vi "BCD码至十进制转换.vi"(9 "低位":u16 format="%x", 11 "高位":u16 format="%x") -> (2 "十进制数":u16)   [LabVIEW 2010]
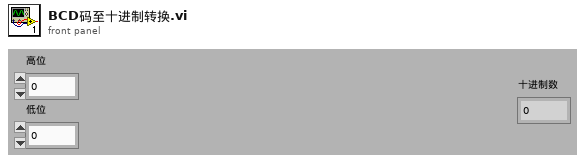
[diagram p1: front panel]
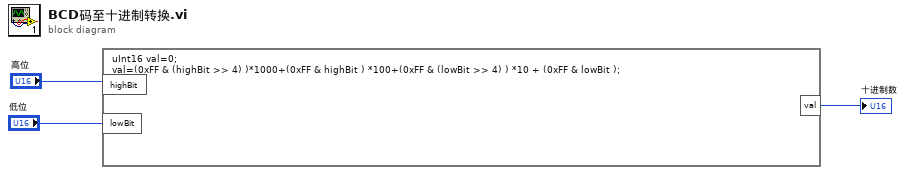
[diagram p0: block diagram]
diagram:
  n1 = formula code="uInt16 val=0;\nval=(0xFF & (highBit >> 4) )*1000+(0xFF & highBit ) *100+(0xFF & (lowBit >> 4) ) *10 + (0xFF & lowBit );"("highBit"="高位", "lowBit"="低位") -> ("val"=→"十进制数":u16)
